vi "idn.vi"(0 "HGF_DeviceBase":refnum<class "HGF_DeviceBase.lvclass">, 5 "error in (no error)":errorcluster) -> (10 "nodeName":string, 11 "identifiationString":string, 12 "resourceString":string, 13 "additionalInfo":string, 14 "dup HGF_DeviceBase":refnum<class "HGF_DeviceBase.lvclass">, 15 "driverRevision":string="unknown", 16 "firmwareRevision":string="unknown", 17 "vendor":string="unknown", 18 "model":string="unknown", 19 "error out":errorcluster)   [LabVIEW 2014, in "HGF_DeviceBaseClasses.lvlib" / "HGF_DeviceBase.lvclass"]
doc: "This VI queries the current instrument firmware revision and instrument driver revision.\n\nFor detailed driver information including modification history, refer to the Readme file.\n\n<b>Hint:</b> This is a dynamic dispatch VI to be implemented by child classes."
uses:
  HGF_DeviceBase.lvclass
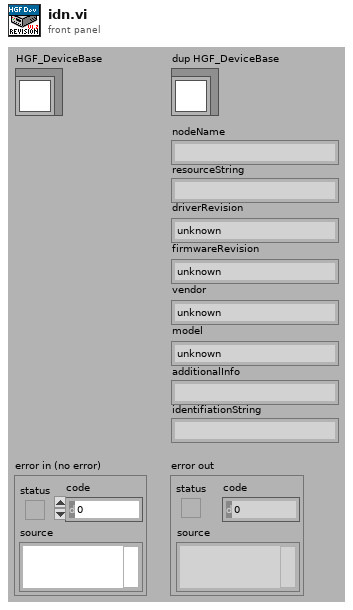
[diagram p1: front panel]
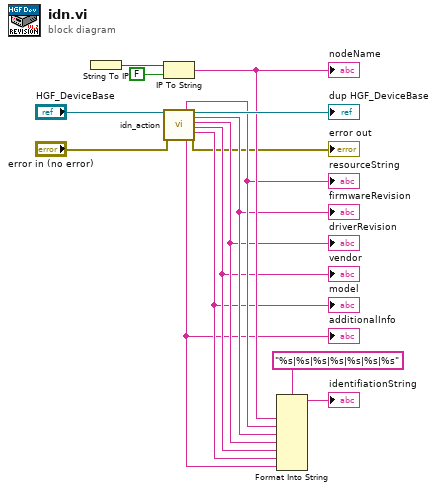
[diagram p0: block diagram]
diagram:
  n1 = String To IP() -> (0:w15:u32)  [unwired: 1 out]
  n2 = IP To String(1:FALSE ("dot notation? (F)"), 2:w15) -> (0:w11:string)
  "nodeName" <- w11
  n3 = call-dynamic "idn_action.vi"("HGF_DeviceBase"="HGF_DeviceBase", "error in (no error)"="error in (no error)") -> ("resourceString"=w10:string, "additionalInfo"=w5:string, "dup HGF_DeviceBase"=→"dup HGF_DeviceBase":refnum<class "HGF_DeviceBase.lvclass">, "driverRevision"=w9:string, "firmwareRevision"=w8:string, "vendor"=w7:string, "model"=w6:string, "error out"=→"error out":errorcluster)  [unwired: 10 out]
  "driverRevision" <- w8
  "firmwareRevision" <- w9
  "vendor" <- w7
  "model" <- w6
  "resourceString" <- w10
  "additionalInfo" <- w5
  n4 = Format Into String(format string="%s|%s|%s|%s|%s|%s|%s", w11, w10, w9, w8, w7, w6, w5) -> (resulting string=→"identifiationString":string)  [unwired: 2 in, 1 out]
